vi "Read Texture Array.vi"(11 "TEXTURES Lump":u8[](array[numeric])) -> (2 "Texture Names Array":string[](array[string]), 3 "Textures array":T1[](array[typedef]))   [LabVIEW 2017]
uses:
  TextureList.ctl
  PatchList.ctl
  <vilib>/Utility/error.llb/Search and Replace Pattern.vi
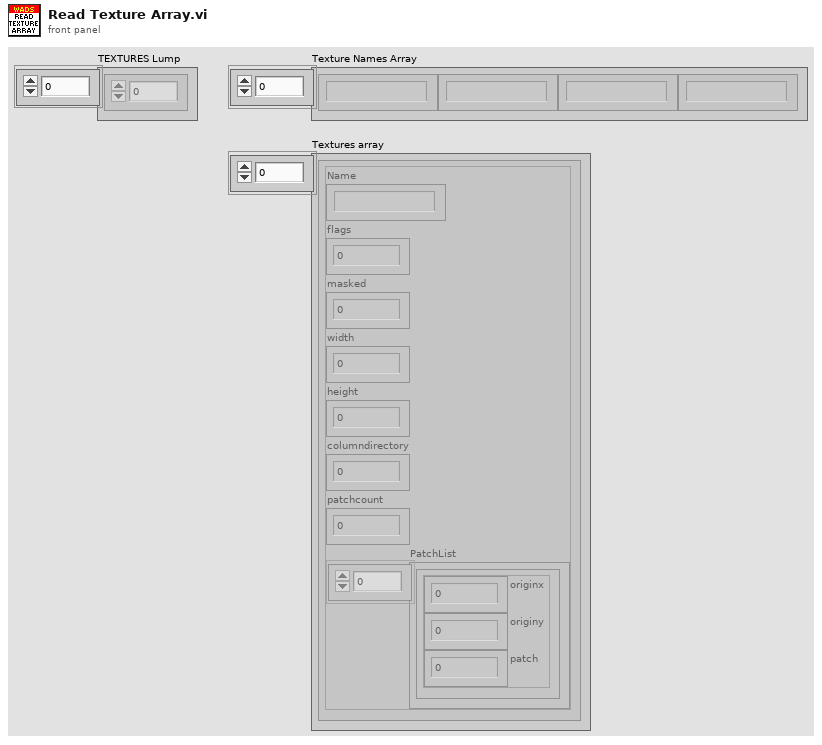
[diagram p1: front panel]
types:
  T1 = typedef "TextureList.ctl" = cluster{"Name":string, "flags":u16, "masked":i16, "width":i16, "height":i16, "columndirectory":u32, "patchcount":i16, "PatchList":T2[]}
  T2 = typedef "PatchList.ctl" = cluster{"originx":i16, "originy":i16, "patch":i16}
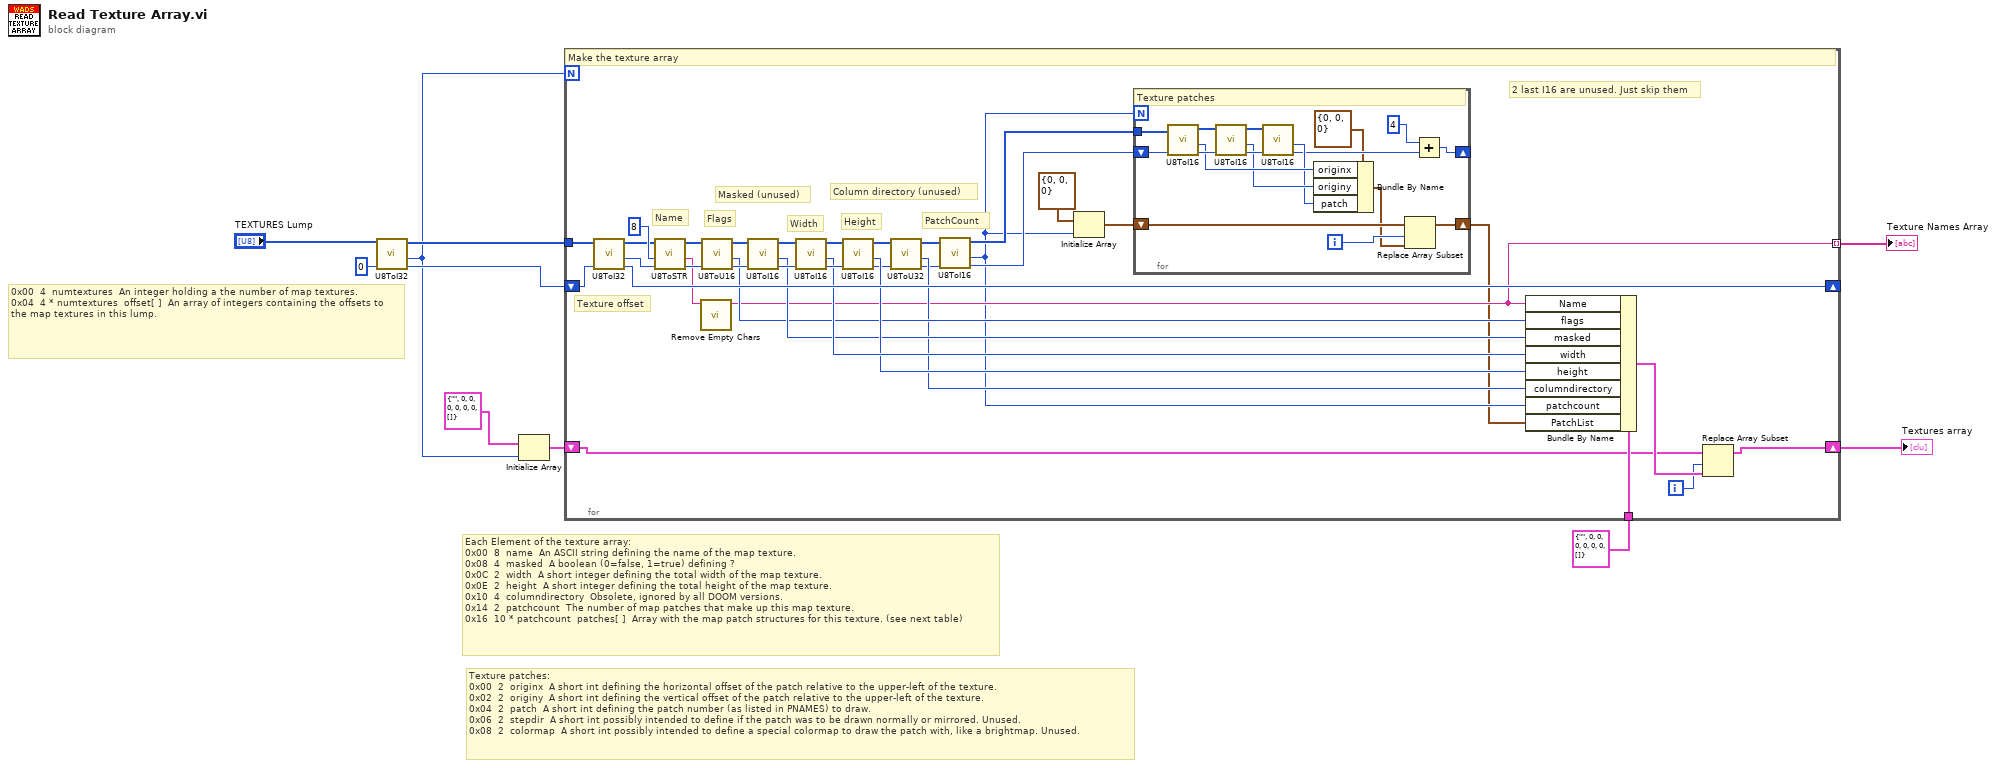
[diagram p0: block diagram]
diagram:
  # "Texture patches:\n0x00 \t2 \toriginx \tA short int defining the horizontal offset of the patch relative to the upper-left of the texture.\n0x02 \t2 \toriginy \tA short int defining the vertical offset of the patch relative to the upper-left of the texture.\n0x04 \t2 \tpatch \tA short int defining the patch number (as listed in PNAMES) to draw.\n0x06 \t2 \tstepdir \tA short int possibly intended to define if the patch was to be drawn normally or mirrored. Unused.\n0x08 \t2 \tcolormap \tA short int possibly intended to define a special colormap to draw the patch with, like a brightmap. Unused."
  # "Each Element of the texture array:\n0x00 \t8 \tname \tAn ASCII string defining the name of the map texture.\n0x08 \t4 \tmasked \tA boolean (0=false, 1=true) defining ?\n0x0C \t2 \twidth \tA short integer defining the total width of the map texture.\n0x0E \t2 \theight \tA short integer defining the total height of the map texture.\n0x10 \t4 \tcolumndirectory \tObsolete, ignored by all DOOM versions.\n0x14 \t2 \tpatchcount \tThe number of map patches that make up this map texture.\n0x16 \t10 * patchcount \tpatches[ ] \tArray with the map patch structures for this texture. (see next table)"
  # "0x00 \t4 \tnumtextures \tAn integer holding a the number of map textures.\n0x04 \t4 * numtextures \toffset[ ] \tAn array of integers containing the offsets to the map textures in this lump."
  n1 = call "U8ToI32.vi"("Index"=u32 0, "Input U8 Array"="TEXTURES Lump") -> ("Index+4"=w4:u32, "Output I32"=w1:i32, "Output U8 Array"=w8:u8[])  [unwired: 3 in]
  n2 = Initialize Array(T1 {"Name"="", "flags"=0, "masked"=0, "width"=0, "height"=0, "columndirectory"=0, "patchcount"=0, "PatchList"=[]}, w1) -> (w3:T1[])
  n3 = for {
    N: w1 -> [_]
    tunnel: w8 -> [w46]
    shift-right: [w44] -> _
    shift-left: w4 -> [w45]
    tunnel: T1 {"Name"="", "flags"=0, "masked"=0, "width"=0, "height"=0, "columndirectory"=0, "patchcount"=0, "PatchList"=[]} -> [w37]
    tunnel: [w20] -> w10 mode=indexing
    shift-right: [w16] -> w2
    shift-left: w3 -> [w17]
    i -> [w15]
    # "2 last I16 are unused. Just skip them"
    # "Texture offset"
    # "Column directory (unused)"
    # "Masked (unused)"
    # "PatchCount"
    # "Height"
    # "Width"
    # "Flags"
    # "Name"
    # "Make the texture array"
    n4 = call "U8ToI32.vi"("Index"=w45, "Input U8 Array"=w46) -> ("Index+4"=w44:u32, "Output I32"=w41:i32, "Output U8 Array"=w42:u8[])  [unwired: 3 in]
    n5 = call "U8ToSTR.vi"("Index"=w41, "Count"=8, "Input U8 Array"=w42) -> ("Index+Count"=w40:u32, "Output String"=w21:string, "Output U8 Array"=w19:u8[])  [unwired: 2 in]
    n6 = call "Remove Empty Chars.vi"("String with \\00"=w21) -> ("String without \\00"=w20:string)  [unwired: 10 in]
    n7 = call "U8ToU16.vi"("Index"=w40, "Input U8 Array"=w19) -> ("Index+2"=w33:u32, "Output U16"=w29:u16, "Output U8 Array"=w34:u8[])  [unwired: 3 in]
    n8 = call "U8ToI16.vi"("Index"=w33, "Input U8 Array"=w34) -> ("Index+2"=w31:u32, "Output I16"=w30:i16, "Output U8 Array"=w32:u8[])  [unwired: 3 in]
    n9 = call "U8ToI16.vi"("Index"=w31, "Input U8 Array"=w32) -> ("Index+2"=w39:u32, "Output I16"=w36:i16, "Output U8 Array"=w38:u8[])  [unwired: 3 in]
    n10 = call "U8ToI16.vi"("Index"=w39, "Input U8 Array"=w38) -> ("Index+2"=w27:u32, "Output I16"=w35:i16, "Output U8 Array"=w28:u8[])  [unwired: 3 in]
    n11 = call "U8ToU32.vi"("Index"=w27, "Input U8 Array"=w28) -> ("Index+4"=w25:u32, "Output U32"=w26:u32, "Output U8 Array"=w24:u8[])  [unwired: 3 in]
    n12 = call "U8ToI16.vi"("Index"=w25, "Input U8 Array"=w24) -> ("Index+2"=w22:u32, "Output I16"=w14:i16, "Output U8 Array"=w23:u8[])  [unwired: 3 in]
    n13 = Initialize Array(T2 {"originx"=0, "originy"=0, "patch"=0} ("PatchList"), w14) -> (w12:T2[])
    n14 = for {
      N: w14 -> [_]
      tunnel: w23 -> [w58]
      shift-right: [w53] -> _
      shift-left: w22 -> [w59]
      shift-right: [w51] -> w11
      shift-left: w12 -> [w50]
      i -> [w49]
      # "Texture patches"
      n15 = call "U8ToI16.vi"("Index"=w59, "Input U8 Array"=w58) -> ("Index+2"=w63:u32, "Output I16"=w57:i16, "Output U8 Array"=w62:u8[])  [unwired: 3 in]
      n16 = call "U8ToI16.vi"("Index"=w63, "Input U8 Array"=w62) -> ("Index+2"=w60:u32, "Output I16"=w56:i16, "Output U8 Array"=w61:u8[])  [unwired: 3 in]
      n17 = call "U8ToI16.vi"("Index"=w60, "Input U8 Array"=w61) -> ("Index+2"=w54:u32, "Output I16"=w55:i16)  [unwired: 3 in, 1 out]
      n18 = Bundle By Name(cluster=T2 {"originx"=0, "originy"=0, "patch"=0} ("PatchList"), "originx"=w57, "originy"=w56, "patch"=w55) -> (w47:T2)
      n19 = Replace Array Subset(array=w50, new element=w47, index=w49) -> (w51:T2[])
      n20 = Add(x=u32 4 ("Index"), y=w54) -> (x+y=w53:u32)
    }
    n21 = Bundle By Name(cluster=w37, "Name"=w20, "flags"=w29, "masked"=w30, "width"=w36, "height"=w35, "columndirectory"=w26, "patchcount"=w14, "PatchList"=w11) -> (w18:T1)
    n22 = Replace Array Subset(array=w17, new element=w18, index=w15) -> (w16:T1[])
  }
  "Texture Names Array" <- w10
  "Textures array" <- w2
